vi "EI Example (A).vi"() -> ()   [LabVIEW 2011]
uses:
  C:/Program Files/Metrohm Autolab/Autolab SDK 1.10/EcoChemie.Autolab.Sdk.dll
  EcoChemie.Autolab.Sdk.dll
panel:
  out "EI status supported for":string[](array[string])
  out "CurrentRange":i32(ring) items=["CR07_1A"=0, "CR06_10A"=1, "CR01_100A"=2, "CR00_1000A"=3, "CR05_20A"=20, "CR04_40A"=40, "CR03_50A"=60, "CR02_80A"=80, "CR19_1pA"=-12, "CR18_10pA"=-11, "CR17_100pA"=-10, "CR16_1nA"=-9, "CR15_10nA"=-8, "CR14_100nA"=-7, "CR13_1uA"=-6, "CR12_10uA"=-5, "CR11_100uA"=-4, "CR10_1mA"=-3, "CR09_10mA"=-2, "CR08_100mA"=-1]
  out "Bandwidth":i32(ring) items=["UltraHigh_Speed", "High_Speed", "High_Stability"]
  out "Mode":i32(ring) items=["Potentiostatic", "Galvanostatic"]
  out "Setpoint":dbl
  out "error out":errorcluster
  in  "stop":bool
  out "IsConnected":bool
  in  "Hardware Setup File":path
  in  "Embedded Exe File":path
  out "Oscillation":bool
  out "Current":dbl
  out "Potential":dbl
  out "PotentialOverload":bool
  out "TemperatureOverload":bool
  out "CurrentOverload":bool
  out "ManualCellSwitch":bool
  out "Cell":bool
  in  "Setpoint":dbl
  in  "Current Range":i32(ring)=-3 items=["CR07_1A"=0, "CR06_10A"=1, "CR01_100A"=2, "CR00_1000A"=3, "CR05_20A"=20, "CR04_40A"=40, "CR03_50A"=60, "CR02_80A"=80, "CR19_1pA"=-12, "CR18_10pA"=-11, "CR17_100pA"=-10, "CR16_1nA"=-9, "CR15_10nA"=-8, "CR14_100nA"=-7, "CR13_1uA"=-6, "CR12_10uA"=-5, "CR11_100uA"=-4, "CR10_1mA"=-3, "CR09_10mA"=-2, "CR08_100mA"=-1]
  in  "Cell On/Off":i32(ring) items=["Off", "On"]
  in  "Bandwidth":i32(ring)=2 items=["UltraHigh_Speed", "High_Speed", "High_Stability"]
  in  "Mode":i32(ring) items=["Potentiostatic", "Galvanostatic"]
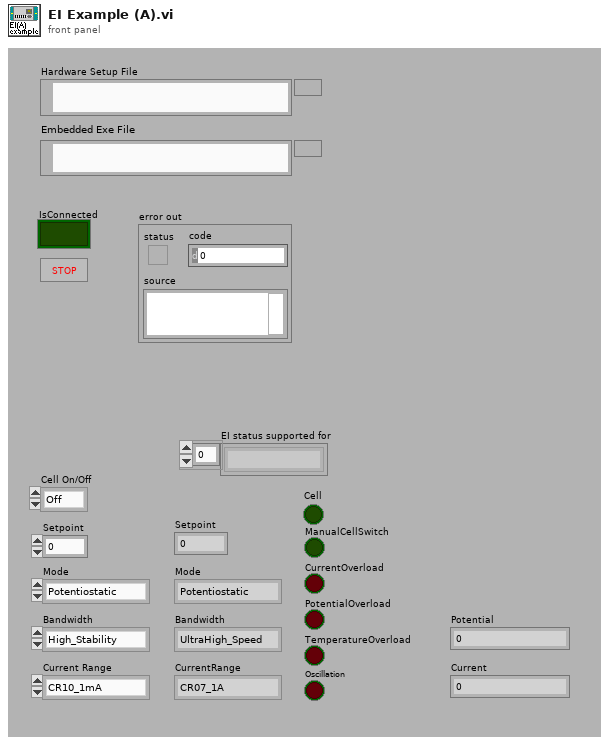
[diagram p1: front panel]
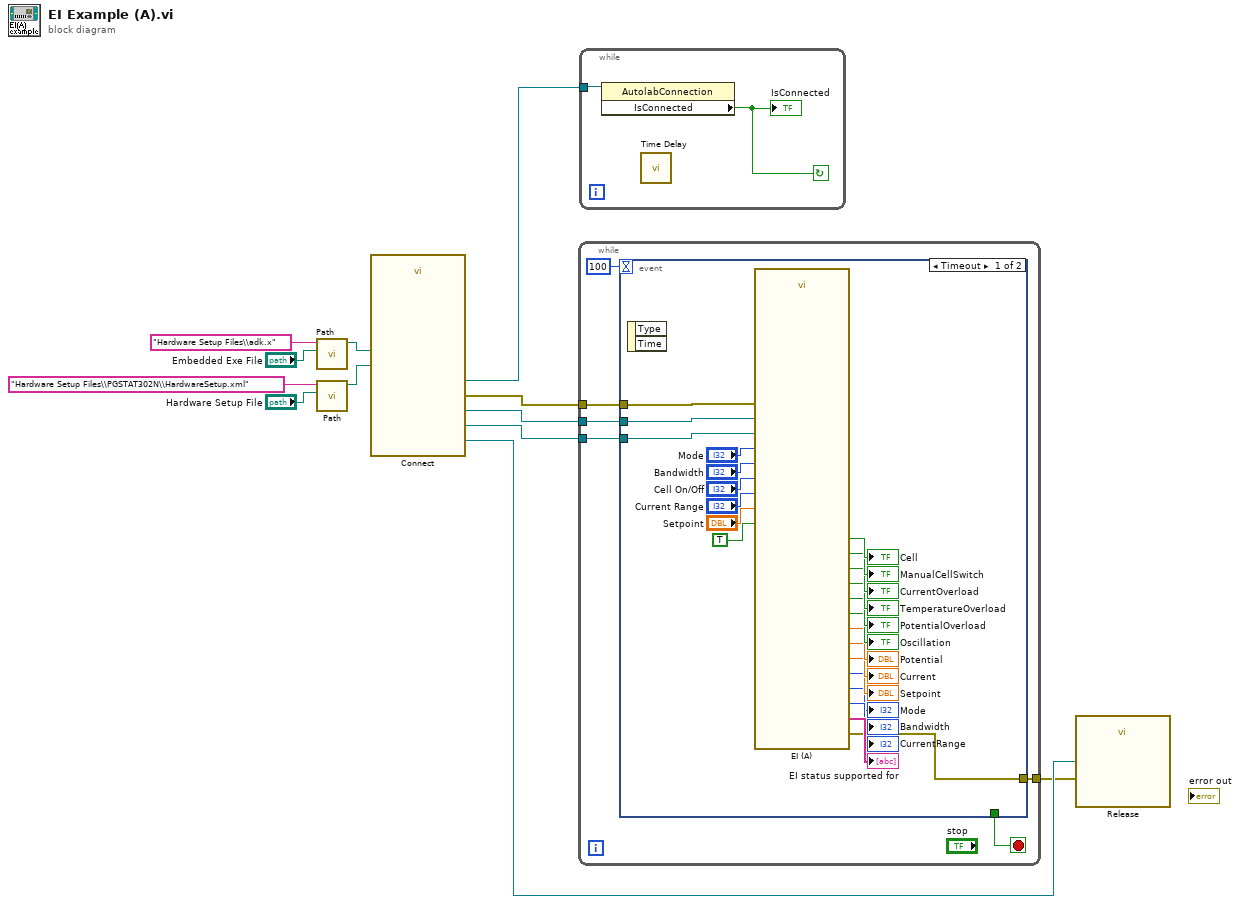
[diagram p0: block diagram]
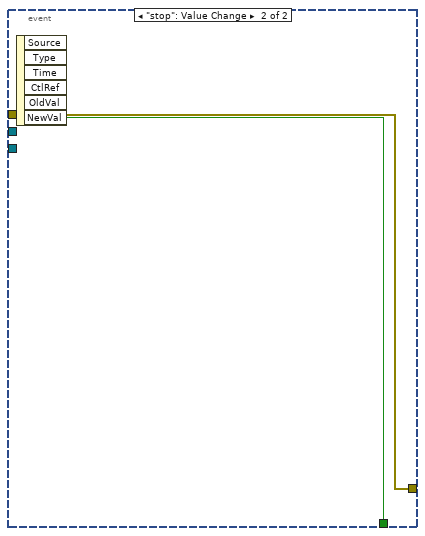
[diagram p2: hidden frame]
diagram:
  n1 = call "Path.vi"("File"="Embedded Exe File", "name or relative path"="Hardware Setup Files\\adk.x") -> ("appended path"=w1:path)  [unwired: 9 in]
  n2 = call "Path.vi"("File"="Hardware Setup File", "name or relative path"="Hardware Setup Files\\PGSTAT302N\\HardwareSetup.xml") -> ("appended path"=w2:path)  [unwired: 9 in]
  n3 = call "Connect.vi"("Embedded Exe File"=w1, "Hardware Setup File"=w2) -> ("Sampler"=w10:refnum<k24>, "AutolabConnection"=w12:refnum<k24>, "instrument"=w8:refnum<k24>, "Ei"=w9:refnum<k24>, "error out"=w11:errorcluster)  [unwired: 6 in, 3 out]
  n4 = while {
    tunnel: w11 -> [w18]
    tunnel: w10 -> [w17]
    tunnel: w9 -> [w16]
    tunnel: [w15] -> w7
    stop <- w13 stop-if-true
    n5 = event shown="[0] Timeout" {
      selector: _ -> [_ _]
      dyn-events: _ -> [_ _]
      timeout: 100 -> [_ _]
      tunnel: w18 -> [w41 w43]
      tunnel: w17 -> [w40 _]
      tunnel: w16 -> [w39 _]
      tunnel: [w19 w43] -> w15
      tunnel: [_ w42] -> w13
      event Timeout {
        n6 = event-data() -> ()  [unwired: 1 in, 2 out]
        n7 = call "EI (A).vi"("Sampler"=w40, "Ei"=w39, "CellOnOff"="Cell On/Off", "Setpoint"="Setpoint", "Bandwidth"="Bandwidth", "CurrentRange"="Current Range", "Mode"="Mode", "error in (no error)"=w41, "Disable Sampler"=TRUE) -> ("Cell"=→"Cell":bool, "PotentialOverload"=→"PotentialOverload":bool, "ManualCellSwitch"=→"ManualCellSwitch":bool, "TemperatureOverload"=→"TemperatureOverload":bool, "CurrentOverload"=→"CurrentOverload":bool, "Oscillation"=→"Oscillation":bool, "Setpoint"=→"Setpoint":dbl, "Bandwidth"=→"Bandwidth":i32, "CurrentRange"=→"CurrentRange":i32, "Mode"=→"Mode":i32, "EI status supported for"=→"EI status supported for":string[], "Potential"=→"Potential":dbl, "Current"=→"Current":dbl, "error out"=w19:errorcluster)  [unwired: 5 in]
      }
      event "stop": Value Change {
        n8 = event-data() -> ("NewVal"=w42:bool)  [unwired: 1 in, 5 out]
      }
    }
  }
  n9 = while {
    tunnel: w12 -> [w45]
    stop <- w44 continue-if-true
    n10 = property class="AutolabConnection"(reference=w45) -> ("IsConnected"=w44:bool)  [unwired: 1 in, 2 out]
    "IsConnected" <- w44
    n11 = call "Time Delay"() -> ()  [unwired: 11 in, 1 out]
  }
  n12 = call "Release.vi"("error in (no error)"=w7, "Instrument"=w8) -> ()  [unwired: 9 in, 1 out]
